vi "QwtPlot.vi"(5 "parent":refnum<class "QWidget.lvclass">, 8 "Error In":errorcluster, 10 "title":string, 11 "Post-Bundled Subclass":refnum<class "QwtPlot.lvclass">) -> (0 "Error Out":errorcluster, 3 "New QwtPlot":refnum<class "QwtPlot.lvclass">)   [LabVIEW 2014, in "QwtPlot.lvclass"]
doc: "LabVIEW-specific documentation is not yet available. See <b>https://qwt.sourceforge.io/class_qwt_plot.html#QwtPlot</b>"
uses:
  QwtPlot.lvclass
  Qt Widgets/QWidget/QWidget.lvclass
  LQ Core/LQCoreEngine/_Internal/LQIdentity Registry Action.ctl
  LQ Core/LQIdentity/LQIdentity.lvclass/LQIdentity.ctl
  LQ Core/LQCoreEngine/LQCoreEngine.lvclass
  LQ Core/LQ Core.lvlib
  LQ Core/LQIdentity/LQIdentity.lvclass
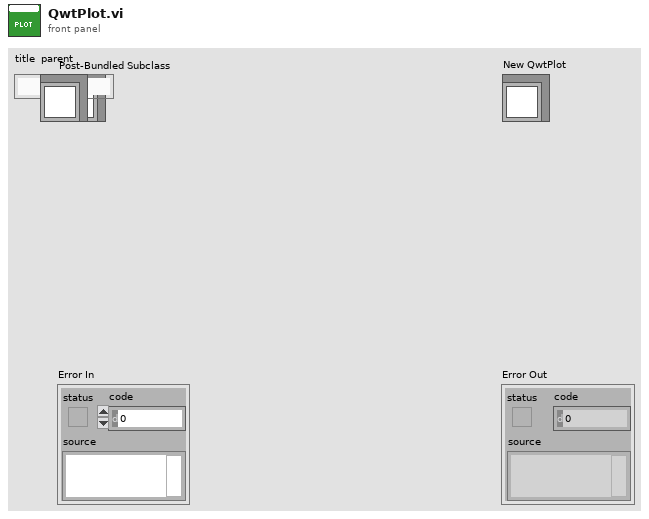
[diagram p1: front panel]
types:
  T1 = typedef "LQ Core.lvlib/LQCoreEngine.lvclass/LQIdentity Registry Action.ctl" = enum16{"Init", "Register LQIdentity", "Get LQIdentity Info", "Deregister LQIdentity"}
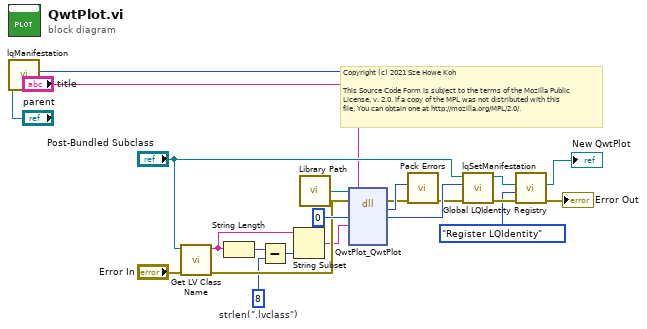
[diagram p0: block diagram]
diagram:
  w7 = 8  # strlen(".lvclass")
  # "Copyright (c) 2021 Sze Howe Koh\n\nThis Source Code Form is subject to the terms of the Mozilla Public\nLicense, v. 2.0. If a copy of the MPL was not distributed with this\nfile, You can obtain one at http://mozilla.org/MPL/2.0/."
  n1 = call "lqManifestation.vi"("LQIdentity in"="parent") -> ("Manifestation"=w1:u64)  [unwired: 9 in, 1 out]
  n2 = call <vilib>:"Get LV Class Name.vi"("error in (no error)"="Error In", "object"="Post-Bundled Subclass") -> ("error out"=w9:errorcluster, "class name"=w5:string)  [unwired: 8 in]
  n3 = String Length(string=w5) -> (length=w8:i32)
  n4 = Subtract(x=w8, y=w7) -> (x-y=w6:i32)
  n5 = String Subset(string=w5, length (rest)=w6) -> (substring=w4:string)  [unwired: 1 in]
  n6 = call "Library Path.vi"() -> ("Library Path"=w20:path)
  n7 = dll-call lib="?" fn="QwtPlot_QwtPlot"(path in=w20, error in=w9, "_retVal"=u64 0 ("_instance"), "_className"=w4, "title"="title", "parent"=w1) -> (error out=w18:errorcluster, w19:i32, "_retVal"=w21:u64)  [unwired: 4 in, 1 out]
  n8 = call "Pack Errors.vi"("Error In"=w18, "Error Code"=w19) -> ("Error Out"=w17:errorcluster)  [unwired: 9 in]
  n9 = call "lqSetManifestation.vi"("Error In"=w17, "Manifestation"=w21, "LQIdentity in"="Post-Bundled Subclass") -> ("Error Out"=w15:errorcluster, "LQIdentity out"=w16:refnum<class "QwtPlot.lvclass">)  [unwired: 7 in]
  n10 = call "Global LQIdentity Registry.vi"("Error In"=w15, "Registry Action"=LQIdentity_Registry_Action."Register LQIdentity", "LQIdentity Info In"=w16) -> ("Error Out"=→"Error Out":errorcluster, "LQIdentity Info Out"=→"New QwtPlot":refnum<class "QwtPlot.lvclass">)  [unwired: 7 in]
